vi "InitializeMission.vi"(4 "Tolerance (m)":dbl, 5 "Done":bool, 6 "Timeout (s)":dbl=-1.0, 7 "Duration (s)":dbl=-1.0, 8 "Error In":errorcluster, 9 "Points of Interest":T1[](array[typedef]) {"North" format="%#_10f"; "East" format="%#_8f"}, 10 "Mission Type":T2, 11 "GenericMission in":refnum<class "GenericMission.lvclass">) -> (0 "Error Out":errorcluster, 3 "GenericMission out":refnum<class "GenericMission.lvclass">)   [LabVIEW 2013, in "GenericMission.lvclass"]
doc: "This VI initializes a mission. Mission Type, Points of Interest, and Tolerance are required, and timeout and duration are both optional."
uses:
  GenericMission.lvclass
  Data/TypeDefs/MissionTypeControl.ctl
  Data/TypeDefs/UTM Location.ctl
  GenericMission.lvclass/GenericMission.ctl
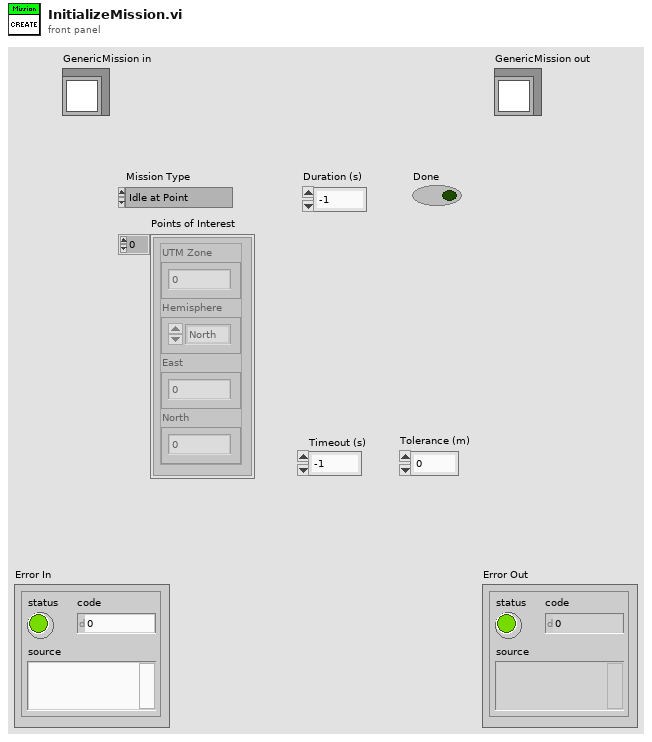
[diagram p1: front panel]
types:
  T1 = typedef "UTM Location.ctl" = cluster{"UTM Zone":dbl, "Hemisphere":enum16{"North", "South"}, "East":dbl, "North":dbl}
  T2 = typedef "MissionTypeControl.ctl" = enum16{"Idle at Point", "Drive to Waypoint", "Round Buoy to Port", "Round Buoy to Starboard", "Pass Between Buoys", "Station Keeping"}
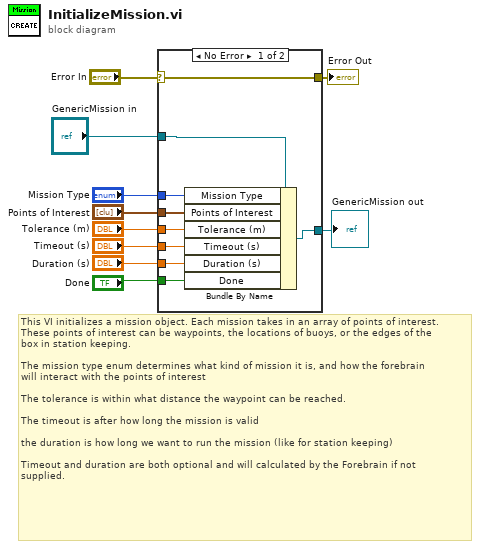
[diagram p0: block diagram]
diagram:
  # "This VI initializes a mission object. Each mission takes in an array of points of interest.\nThese points of interest can be waypoints, the locations of buoys, or the edges of the \nbox in station keeping. \n\nThe mission type enum determines what kind of mission it is, and how the forebrain \nwill interact with the points of interest\n\nThe tolerance is within what distance the waypoint can be reached. \n\nThe timeout is after how long the mission is valid\n\nthe duration is how long we want to run the mission (like for station keeping)\n\nTimeout and duration are both optional and will calculated by the Forebrain if not \nsupplied."
  n1 = case shown="No Error" "Error In" {
    selector: "Error In" -> [w19 w20]
    tunnel: [w19 w20] -> w9
    tunnel: "Mission Type" -> [w18 _]
    tunnel: "Points of Interest" -> [w17 _]
    tunnel: "Tolerance (m)" -> [w16 _]
    tunnel: "Timeout (s)" -> [w15 _]
    tunnel: "Duration (s)" -> [w14 _]
    tunnel: "GenericMission in" -> [w13 w21]
    tunnel: [w12 w21] -> w2
    tunnel: "Done" -> [w11 _]
    frame No Error {
      n2 = Bundle By Name(cluster=w13, "Mission Type"=w18, "Points of Interest"=w17, "Tolerance (m)"=w16, "Timeout (s)"=w15, "Duration (s)"=w14, "Done"=w11) -> (w12:refnum<class "GenericMission.lvclass">)
    }
    frame Error {
    }
  }
  "Error Out" <- w9
  "GenericMission out" <- w2
